vi "WaitStopEPS.vi"(5 "VISA resource name":refnum<visa-resource-name>) -> (0 "Error Status":bool, 1 "Stopped":bool, 2 "VISA resource name out":refnum<visa-resource-name>)   [LabVIEW 2022 SP3]
uses:
  <instrlib>/Newport ESP301/Newport ESP301.lvlib
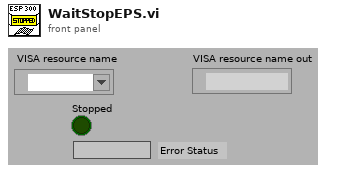
[diagram p1: front panel]
types:
  T1 = cluster{"Axis1 moving":bool, "Axis2 moving":bool, "Axis3 moving":bool, "Axis4 moving":bool, "Motor Power of at least one axis":bool, "Reserved":bool, "Reserved":bool, "Reserved":bool, "Axis5 moving 2":bool, "Axis6 moving 2":bool, "Reserved":bool, "Reserved":bool, "Motor Power of at least one axis":bool, "Reserved":bool, "Reserved":bool, "Reserved":bool}
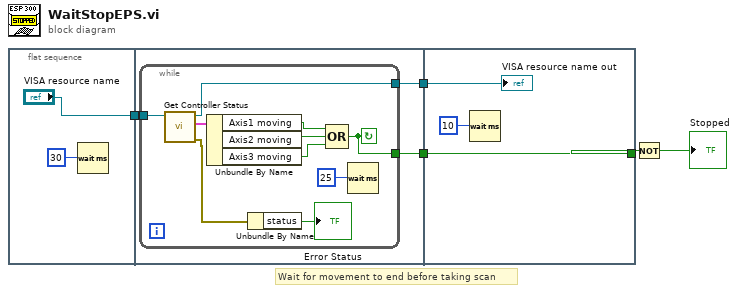
[diagram p0: block diagram]
diagram:
  # "Wait for movement to end before taking scan"
  n1 = flat-sequence {
    tunnel: ["VISA resource name"] -> w2
    tunnel: [w10] -> w4
    tunnel: [w9] -> w3
    tunnel: w2 -> [w8]
    tunnel: [w23] -> w5
    tunnel: w4 -> [w23]
    tunnel: w3 -> [w21]
    frame #0 {
      n2 = Wait (ms)(milliseconds to wait=30) -> ()  [unwired: 1 out]
    }
    frame #1 {
      n3 = while {
        tunnel: [w19] -> w10
        tunnel: [w13] -> w9
        tunnel: w8 -> [w12]
        stop <- w19 continue-if-true
        n4 = call <instrlib>:"Get Controller Status.vi"("VISA resource name"=w12) -> ("error out"=w15:errorcluster, "Controller Status"=w18:T1, "VISA resource name out"=w13:refnum<visa-resource-name>)  [unwired: 4 in]
        n5 = Unbundle By Name(w18) -> ("Axis1 moving"=w17:bool, "Axis2 moving"=w16:bool, "Axis3 moving"=w11:bool)
        n6 = Unbundle By Name(w15) -> ("status"=→"Error Status":bool)
        n7 = Compound Arithmetic op=OR(w17, w16, w11) -> (w19:bool)
        n8 = Wait (ms)(milliseconds to wait=25) -> ()  [unwired: 1 out]
      }
    }
    frame #2 {
      n9 = Wait (ms)(milliseconds to wait=10) -> ()  [unwired: 1 out]
      "VISA resource name out" <- w21
    }
  }
  n10 = Not(x=w5) -> (.not. x?=→"Stopped":bool)
